vi "Mulit-Clients Example.vi"   [LabVIEW 2020]
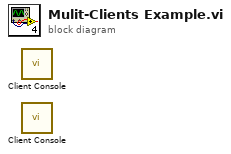
[diagram p0: block diagram]
diagram:
  n1 = call "Client Console.vi"() -> ()  [unwired: 12 in]
  n2 = call "Client Console.vi"() -> ()  [unwired: 12 in]
